vi "number2Color.vi"() -> ()   [LabVIEW 2009, in "run.lvlib"]
uses:
  run.lvlib
panel:
  out "HEX Color":u32=16776960 format="%x"
  in  "Color":u32(colorbox)
  in  "HEX Color: RRGGBB":u32=16776960 format="%x"
  out "Color Box":u32(colorbox)
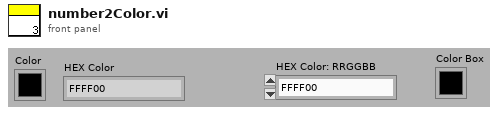
[diagram p1: front panel]
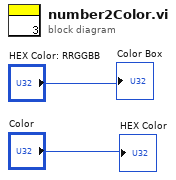
[diagram p0: block diagram]
diagram:
  "Color Box" <- "HEX Color: RRGGBB"
  "HEX Color" <- "Color"
